vi "send_command.vi"(6 "Ampiezza":string, 9 "Step in frequenza":dbl, 10 "Costante":dbl, 11 "f_start":dbl) -> (1 "out Comando frequenza":string, 2 "out Comando ampiezza":string, 3 "Comando ampiezza":string, 4 "Frequenza corrente":dbl, 5 "out Frequenza corrente":dbl, 7 "Comando frequenza":string)   [LabVIEW 2021]
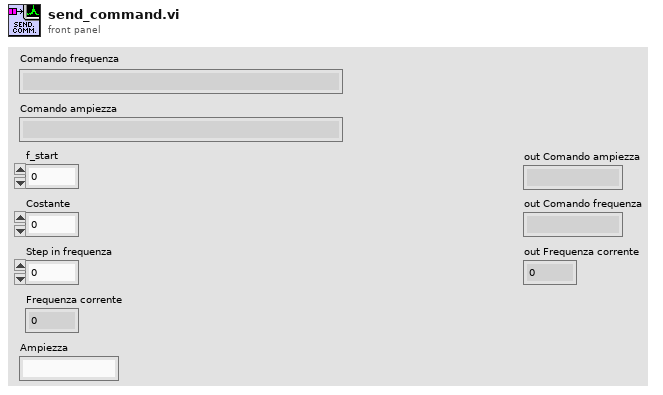
[diagram p1: front panel]
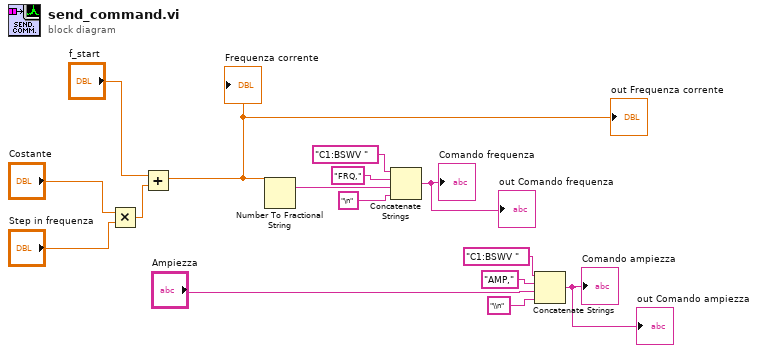
[diagram p0: block diagram]
diagram:
  n1 = Multiply(x="Costante", y="Step in frequenza") -> (x*y=w13:dbl)
  n2 = Add(x="f_start", y=w13) -> (x+y=w15:dbl)
  "Frequenza corrente" <- w15
  "out Frequenza corrente" <- w15
  n3 = Number To Fractional String(number=w15) -> (F-format string=w3:string)  [unwired: 3 in]
  n4 = Concatenate Strings("C1:BSWV ", "FRQ,", w3, "\n" ("string")) -> (→"Comando frequenza" →"out Comando frequenza":string)
  n5 = Concatenate Strings("C1:BSWV ", "AMP," ("string"), "Ampiezza", "\\n" ("string")) -> (→"Comando ampiezza" →"out Comando ampiezza":string)
